vi "RunGlue.vi"() -> ()   [LabVIEW 2016]
panel:
  in  "Dry Run":bool
  out "Finished":bool
  in  "Stereo Angle [mrad]":dbl=-26.0
  in  "Module Number":i32=1
  in  "Calibration Directory":path=path "C:/Users/Aerotech/Documents/Zach/Mounting-Module1"
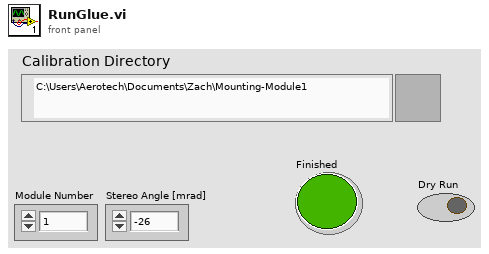
[diagram p1: front panel]
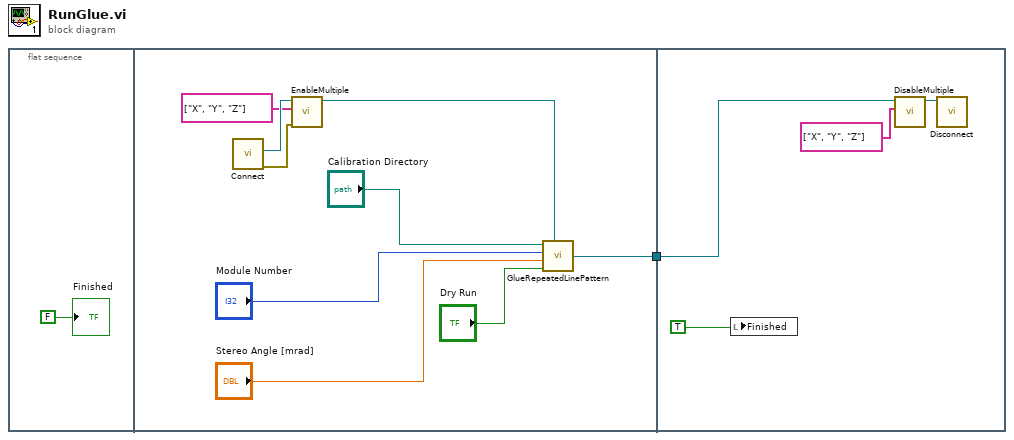
[diagram p0: block diagram]
diagram:
  n1 = flat-sequence {
    tunnel: [w3] -> w1
    tunnel: w1 -> [w12]
    frame #0 {
      "Finished" <- FALSE ("Finished")
    }
    frame #1 {
      n2 = call "Connect.vi"() -> ("error out"=w10:errorcluster, "controller"=w11:refnum<k24>)  [unwired: 10 in]
      n3 = call "EnableMultiple.vi"("error in (no error)"=w10, "axis names"=string[] ["X", "Y", "Z"] ("Axes Names"), "controller in"=w11) -> ("controller out"=w4:refnum<k24>)  [unwired: 7 in, 1 out]
      n4 = call "GlueRepeatedLinePattern.vi"("Controller In"=w4, "Dry Run"="Dry Run", "Stereo Angle [mrad]"="Stereo Angle [mrad]", "Module Number"="Module Number", "Calibration Directory"="Calibration Directory") -> (".NET Refnum out"=w3:refnum<k24>)  [unwired: 1 in]
    }
    frame #2 {
      n5 = local write "Finished"(TRUE ("Dry Run")) -> ()
      n6 = call "DisableMultiple.vi"("axis names"=string[] ["X", "Y", "Z"], "controller in"=w12) -> ("controller out"=w15:refnum<k24>)  [unwired: 8 in, 1 out]
      n7 = call "Disconnect.vi"("controller"=w15) -> ()  [unwired: 10 in, 1 out]
    }
  }
